vi "Configure.vi"(8 "error in (no error)":errorcluster, 10 "Settings in":cluster{"IP Address":string, "Port":u16}, 11 "TCP in":refnum<class "TCP.lvclass">) -> (0 "error out":errorcluster, 3 "TCP out":refnum<class "TCP.lvclass">)   [LabVIEW 2019, in "Protocols.lvlib" / "TCP.lvclass"]
uses:
  TCP.lvclass
  Protocol Parent/Protocol Parent.lvclass
panel:
  in  "Numeric":dbl
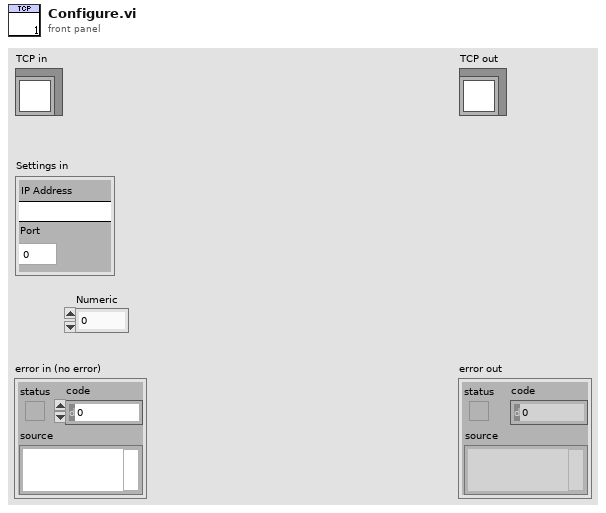
[diagram p1: front panel]
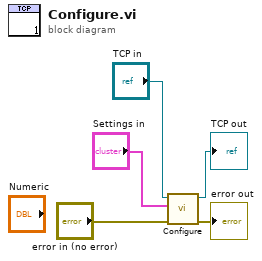
[diagram p0: block diagram]
diagram:
  n1 = call-parent "Configure.vi"("error in (no error)"="error in (no error)", "Settings in"="Settings in", "Protocol Parent in"="TCP in") -> ("error out"=→"error out":errorcluster, "Protocol Parent out"=→"TCP out":refnum<class "TCP.lvclass">)  [unwired: 7 in]
